vi "PID Multi-Channel PID Frame 0.vi"(0 "setpoint":i16, 1 "proportional gain (Kc) (k)":i16, 2 "derivative gain (Kc*Td/Ts) (k)":i16, 5 "PV(k)":i16, 7 "e(k-1)":i16, 9 "PV(k-1)":i16) -> (4 "[e(k)+e(k-1)]/2":i16, 6 "PV(k)":i16, 8 "e(k)":i16, 10 "u_p(k)":i32, 15 "u_d(k)":i32)   [LabVIEW 2017, in "NI_PID_FPGA.lvlib"]
uses:
  <vilib>/addons/control/pid/NI_PID_FPGA.lvlib
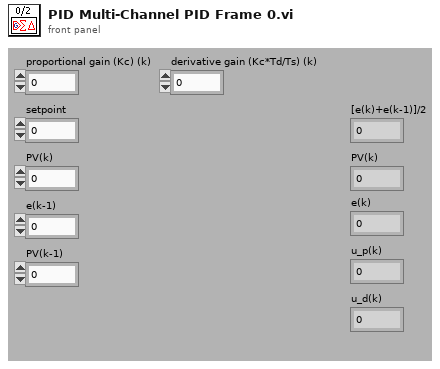
[diagram p1: front panel]
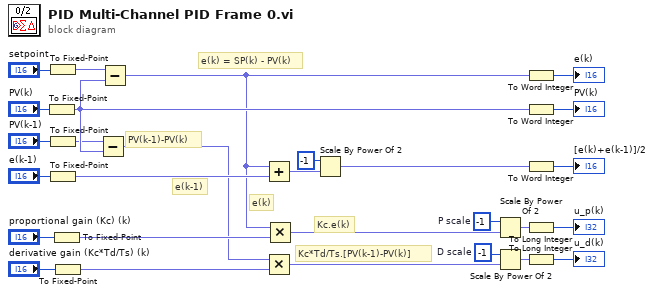
[diagram p0: block diagram]
diagram:
  w24 = i8 -1  # D scale
  w23 = i8 -1  # P scale
  # "PV(k-1)-PV(k)"
  # "Kc*Td/Ts.[PV(k-1)-PV(k)]"
  # "Kc.e(k)"
  # "e(k-1)"
  # "e(k)"
  # "e(k) = SP(k) - PV(k)"
  n1 = To Fixed-Point(number="PV(k)") -> (fixed-point=w21:fxp<+/-,16,16>)  [unwired: 1 in]
  n2 = To Fixed-Point(number="setpoint") -> (fixed-point=w14:fxp<+/-,16,16>)  [unwired: 1 in]
  n3 = To Fixed-Point(number="PV(k-1)") -> (fixed-point=w12:fxp<+/-,16,16>)  [unwired: 1 in]
  n4 = To Fixed-Point(number="e(k-1)") -> (fixed-point=w10:fxp<+/-,16,16>)  [unwired: 1 in]
  n5 = To Fixed-Point(number="proportional gain (Kc) (k)") -> (fixed-point=w8:fxp<+/-,16,16>)  [unwired: 1 in]
  n6 = To Fixed-Point(number="derivative gain (Kc*Td/Ts) (k)") -> (fixed-point=w4:fxp<+/-,16,16>)  [unwired: 1 in]
  n7 = Subtract(x=w12, y=w21) -> (x-y=w5:fxp<+/-,16,16>)
  n8 = Subtract(x=w14, y=w21) -> (x-y=w6:fxp<+/-,16,16>)
  n9 = Add(x=w6, y=w10) -> (x+y=w20:fxp<+/-,17,17>)
  n10 = Multiply(x=w5, y=w4) -> (x*y=w3:fxp<+/-,32,32>)
  n11 = Multiply(x=w6, y=w8) -> (x*y=w19:fxp<+/-,32,32>)
  n12 = Scale By Power Of 2(n=i8 -1, x=w20) -> (x*2^n=w26:fxp<+/-,17,17>)
  n13 = Scale By Power Of 2(n=w23, x=w19) -> (x*2^n=w28:fxp<+/-,32,32>)
  n14 = Scale By Power Of 2(n=w24, x=w3) -> (x*2^n=w27:fxp<+/-,32,32>)
  n15 = To Word Integer(number=w6) -> (16bit integer=→"e(k)":i16)
  n16 = To Word Integer(number=w21) -> (16bit integer=→"PV(k)":i16)
  n17 = To Word Integer(number=w26) -> (16bit integer=→"[e(k)+e(k-1)]/2":i16)
  n18 = To Long Integer(number=w28) -> (32bit integer=→"u_p(k)":i32)
  n19 = To Long Integer(number=w27) -> (32bit integer=→"u_d(k)":i32)
